vi "Turret_Globals.vi"() -> ()   [LabVIEW 2020]
uses:
  Subsystems/Turret/Turret_Cluster.ctl
  Subsystems/Turret/Turret_States.ctl
  <vilib>/Rock Robotics/WPI/ThirdParty/Phoenix-LabVIEW/Motor Controller/Controls/CTRE_Phoenix_MotorControl_ControlMode.ctl
panel:
  out "Turret_Error":dbl=2.0
  out "SWM_Turret_Locked":bool
  in  "Turret_Max_Offset(deg)":dbl=2.0
  in  "Turret_Offset":dbl=2.0
  in  "upper_limit(degrees)":dbl=180.0
  in  "lower_limit(degrees)":dbl=-180.0
  out "Disable_Turret_Safety":bool
  in  "Turret Control Mode":T1 items=["PercentOutput"=0, "Position"=1, "Velocity"=2, "Current"=3, "Follower"=5, "MotionProfile"=6, "MotionMagic"=7, "MotionProfileArc"=10, "Disabled"=15]
  in  "Turret_Spin_Output":dbl
  out "Turret_Locked":bool
  in  "Turret_CANcoder":string="Turret_CANcoder"
  in  "Turret_Spin":string="Turret_Spin"
  in  "Turret_Execute_Notifier":refnum<notifier>
  in  "Turret_Set_Notifier":refnum<notifier>
  in  "Turret_Execute_Ref":string="Turret_Execute_Ref"
  in  "Turret_Set_Ref":string="Turret_Set_Ref"
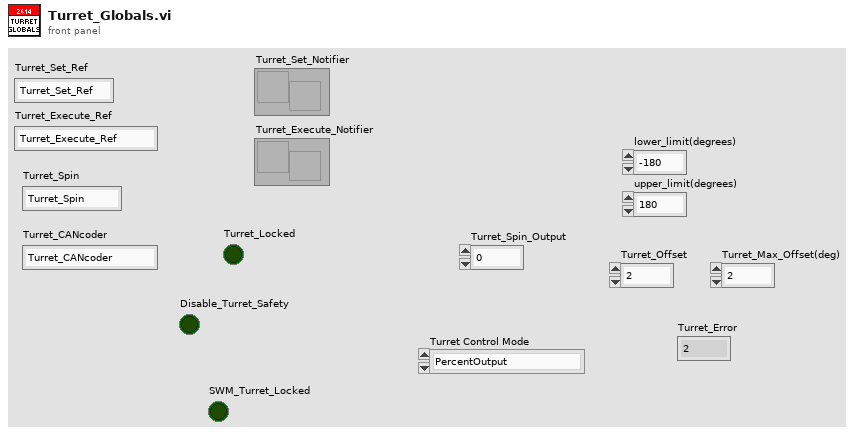
[diagram p1: front panel]
types:
  T1 = typedef "CTRE_Phoenix_MotorControl_ControlMode.ctl" = u16
diagram:
